vi "G#Debugger_GetPublicMethods.vi"(0 "Active Project":refnum<vi>, 1 "ClassName":string, 5 "error in (no error)":errorcluster) -> (15 "Methods":string[](array[string]), 16 "MethodPaths":path[](array[path]), 17 "Item indent":i32[](array[numeric]), 19 "error out":errorcluster)   [LabVIEW 2020, in "G#Debugger.lvlib"]
uses:
  <vilib>/addons/_AddQ/G#Debugger/G#Debugger.lvlib
panel:
  out "Found":bool
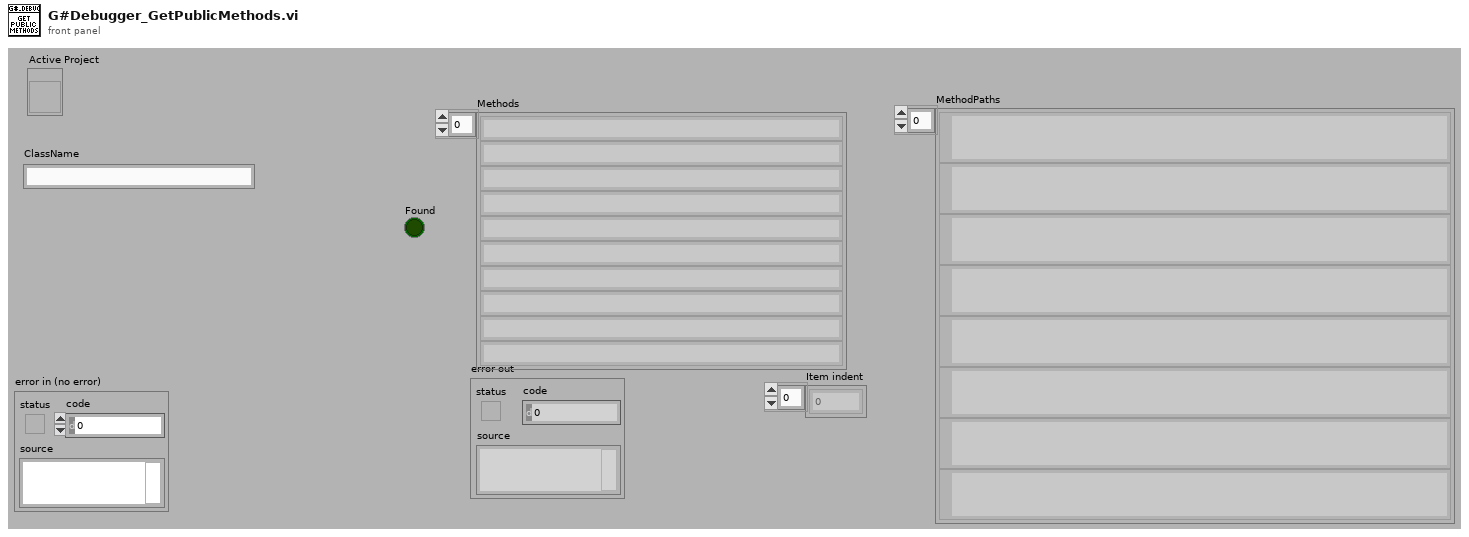
[diagram p1: front panel]
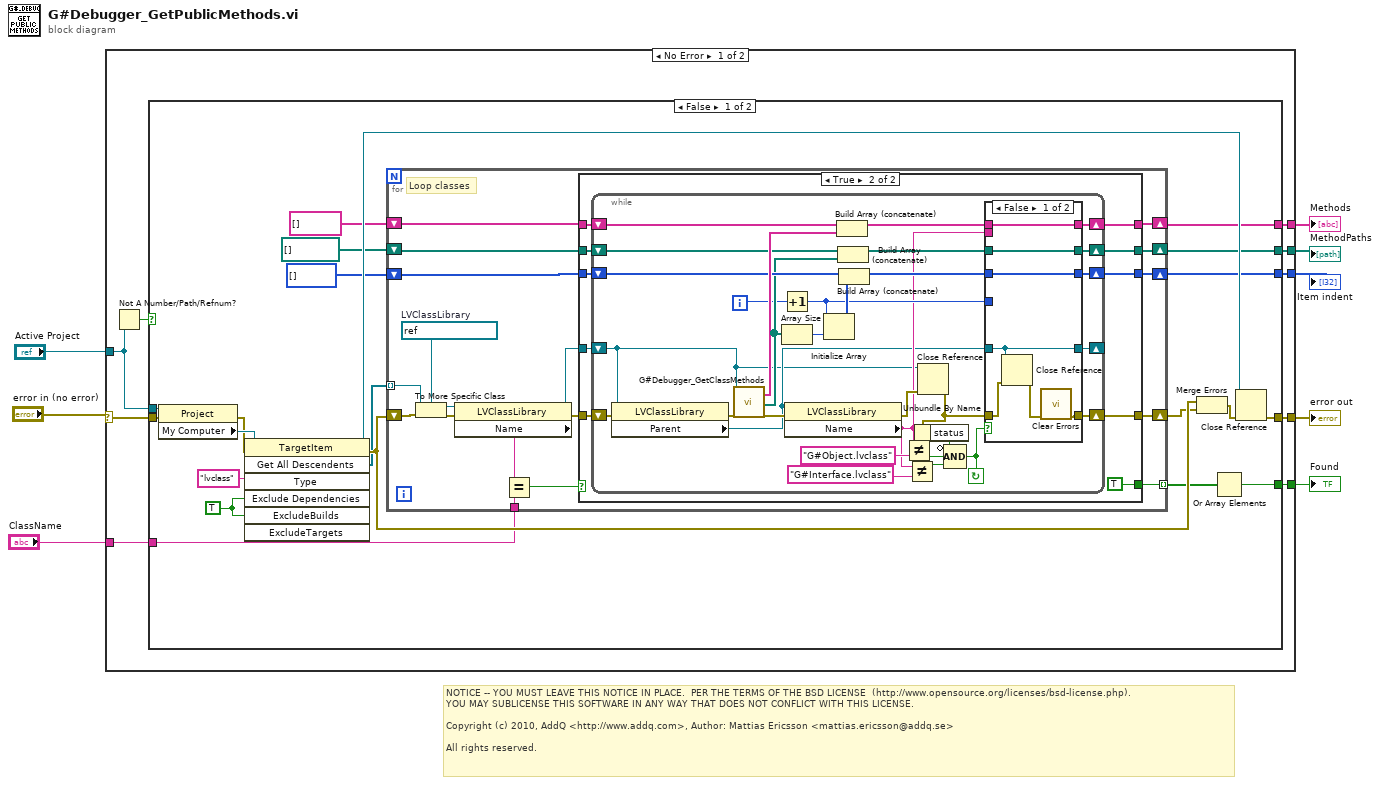
[diagram p0: block diagram]
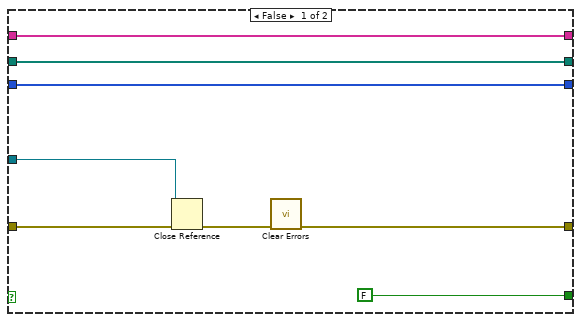
[diagram p2: hidden frame]
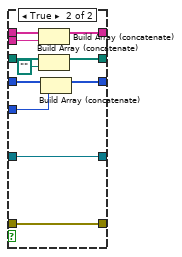
[diagram p3: hidden frame]
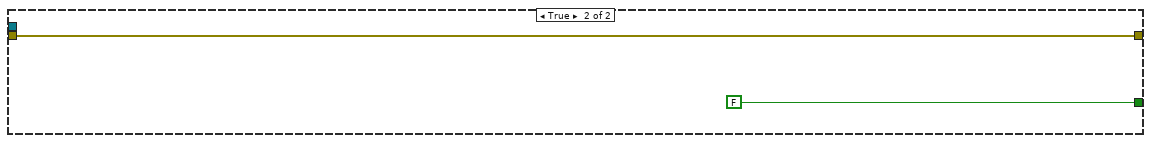
[diagram p4: hidden frame]
diagram:
  # "NOTICE -- YOU MUST LEAVE THIS NOTICE IN PLACE.  PER THE TERMS OF THE BSD LICENSE  (http://www.opensource.org/licenses/bsd-license.php).\nYOU MAY SUBLICENSE THIS SOFTWARE IN ANY WAY THAT DOES NOT CONFLICT WITH THIS LICENSE.\n\nCopyright (c) 2010, AddQ <http://www.addq.com>, Author: Mattias Ericsson <mattias.ericsson@addq.se>\n\nAll rights reserved."
  n1 = case shown="No Error" "error in (no error)" {
    selector: "error in (no error)" -> [w10 w126]
    tunnel: [w9 w126] -> w7
    tunnel: [w17 _] -> w6
    tunnel: [w15 _] -> w5
    tunnel: "ClassName" -> [w12 _]
    tunnel: [w14 _] -> w3
    tunnel: [w13 _] -> w2
    tunnel: "Active Project" -> [w11 _]
    frame No Error {
      n2 = Not A Number/Path/Refnum?(number/path/refnum=w11) -> (NaN/Path/Refnum?=w16:bool)
      n3 = case shown="False" w16 {
        tunnel: w10 -> [w34 w125]
        tunnel: [w26 w125] -> w9
        tunnel: [w20 _] -> w17
        tunnel: w11 -> [w30 _]
        tunnel: [w19 _] -> w15
        tunnel: w12 -> [w29 _]
        tunnel: [w25 FALSE] -> w14
        tunnel: [w18 _] -> w13
        frame False {
          w35 = TRUE ("ExcludeDependencies")
          n4 = property class="Project"(reference=w30, error in=w34) -> (error out=w36:errorcluster, "My Computer"=w38:refnum<vi>)  [unwired: 1 out]
          n5 = invoke class="TargetItem" method="Get All Descendents"(reference=w38, error in=w36, "Type"="lvclass", "Exclude Dependencies"=w35, "ExcludeBuilds"=w35) -> (reference out=w31:refnum<vi>, error out=w33:errorcluster, "All Descendents"=w28:refnum<vi>[])  [unwired: 2 in, 4 out]
          n6 = for {
            shift-right: [w47] -> w27
            shift-left: w33 -> [w56]
            tunnel: w28 -> [w55] mode=indexing
            tunnel: w29 -> [w50]
            tunnel: [w45] -> w24 mode=indexing
            shift-right: [w41] -> w20
            shift-left: string[] [] ("method names") -> [w44]
            shift-right: [w40] -> w19
            shift-left: path[] [] ("method paths") -> [w43]
            shift-right: [w39] -> w18
            shift-left: i32[] [] -> [w42]
            w54 = refnum<vi> refnum  # LVClassLibrary
            # "Loop classes"
            n7 = To More Specific Class(target class=w54, reference=w55, error in=w56) -> (specific class reference=w52:refnum<vi>, error out=w53:errorcluster)
            n8 = property class="LVClassLibrary"(reference=w52, error in=w53) -> (reference out=w48:refnum<vi>, error out=w51:errorcluster, "Name"=w46:string)
            n9 = Equal?(x=w46, y=w50) -> (x = y?=w49:bool)
            n10 = case shown="True" w49 {
              tunnel: w51 -> [w63 w73]
              tunnel: w48 -> [w62 w72]
              tunnel: [w61 w71] -> w41
              tunnel: [w60 w70] -> w40
              tunnel: [w57 w65] -> w47
              tunnel: [FALSE TRUE] -> w45
              tunnel: [w59 w69] -> w39
              tunnel: w44 -> [w61 w68]
              tunnel: w43 -> [w60 w67]
              tunnel: w42 -> [w59 w66]
              frame False {
                n11 = Close Reference(reference=w62, error in (no error)=w63) -> (error out=w58:errorcluster)
                n12 = call <vilib>:"Clear Errors.vi"("error in (no error)"=w58) -> ("error out"=w57:errorcluster)  [unwired: 5 in, 1 out]
              }
              frame True {
                n13 = while {
                  shift-right: [w85] -> _
                  shift-left: w72 -> [w75]
                  shift-right: [w86] -> w65
                  shift-left: w73 -> [w88]
                  shift-right: [w93] -> w71
                  shift-left: w68 -> [w103]
                  shift-right: [w94] -> w70
                  shift-left: w67 -> [w101]
                  shift-right: [w90] -> w69
                  shift-left: w66 -> [w100]
                  i -> [w97]
                  stop <- w79 continue-if-true
                  n14 = property class="LVClassLibrary"(reference=w75, error in=w88) -> (error out=w87:errorcluster, "Parent"=w76:refnum<vi>)  [unwired: 1 out]
                  n15 = call <vilib>:"G#Debugger_GetClassMethods.vi"("LVClassLibrary Refnum"=w75, "error in (no error)"=w87) -> ("method names"=w102:string[], "method paths"=w98:path[], "error out"=w105:errorcluster)  [unwired: 15 in]
                  n16 = Increment(x=w97) -> (x+1=w89:i32)
                  n17 = Array Size(array=w98) -> (size(s)=w99:i32)
                  n18 = property class="LVClassLibrary"(reference=w76, error in=w105) -> (error out=w104:errorcluster, "Name"=w83:string)  [unwired: 1 out]
                  n19 = Initialize Array(w89, w99) -> (w96:i32[])
                  n20 = Build Array (concatenate)(w103, w102) -> (w95:string[])
                  n21 = Build Array (concatenate)(w101, w98) -> (w92:path[])
                  n22 = Build Array (concatenate)(w100, w96) -> (w91:i32[])
                  n23 = Not Equal?(x=w83, y="G#Object.lvclass") -> (x != y?=w80:bool)
                  n24 = Not Equal?(x=w83, y="G#Interface.lvclass") -> (x != y?=w81:bool)
                  n25 = Close Reference(reference=w75, error in (no error)=w104) -> (error out=w78:errorcluster)
                  n26 = Unbundle By Name(w78) -> ("status"=w77:bool)
                  n27 = Compound Arithmetic op=AND(invert w77, w80, w81) -> (w79:bool)
                  n28 = case shown="False" w79 {
                    tunnel: w95 -> [w112 w123]
                    tunnel: w83 -> [_ w122]
                    tunnel: [w111 w118] -> w94
                    tunnel: [w112 w121] -> w93
                    tunnel: w92 -> [w111 w120]
                    tunnel: w91 -> [w110 w117]
                    tunnel: [w110 w116] -> w90
                    tunnel: w89 -> [_ w115]
                    tunnel: w78 -> [w108 w114]
                    tunnel: [w106 w114] -> w86
                    tunnel: w76 -> [w109 w113]
                    tunnel: [w109 w113] -> w85
                    frame False {
                      n29 = Close Reference(reference=w109, error in (no error)=w108) -> (error out=w107:errorcluster)
                      n30 = call <vilib>:"Clear Errors.vi"("error in (no error)"=w107) -> ("error out"=w106:errorcluster)  [unwired: 5 in, 1 out]
                    }
                    frame True {
                      n31 = Build Array (concatenate)(w123, w122) -> (w121:string[])
                      n32 = Build Array (concatenate)(w120, path "") -> (w118:path[])
                      n33 = Build Array (concatenate)(w117, w115) -> (w116:i32[])
                    }
                  }
                }
              }
            }
          }
          n34 = Merge Errors(w33, w27) -> (w32:errorcluster)
          n35 = Or Array Elements(Boolean array=w24) -> (logical OR=w25:bool)
          n36 = Close Reference(reference=w31, error in (no error)=w32) -> (error out=w26:errorcluster)
        }
        frame True {
        }
      }
    }
    frame Error {
    }
  }
  "error out" <- w7
  "Methods" <- w6
  "MethodPaths" <- w5
  "Found" <- w3
  "Item indent" <- w2
